vi "Medicao_anemometro.vi"(8 "Array 2":dbl[](array[numeric]), 9 "Sinalinp":dbl, 10 "Anemometro":dbl, 11 "DadosGraphInp":cluster{"GraphSenoide":i32[], "NivelAlto":bool}) -> (2 "Sinal":dbl, 3 "DadosGraph":cluster{"GraphSenoide":i32[], "NivelAlto":bool})   [LabVIEW 2019]
panel:
  out "Array":i32[](array[numeric])
  out "Anemometro 2":dbl
  in  "XY Graph 2":cluster{"X":dbl, "Y":dbl}[](graph)
  out "y 3":dbl
  out "y 2":dbl
  out "Array 4":dbl[](array[numeric])
  # "3,57812E+8"
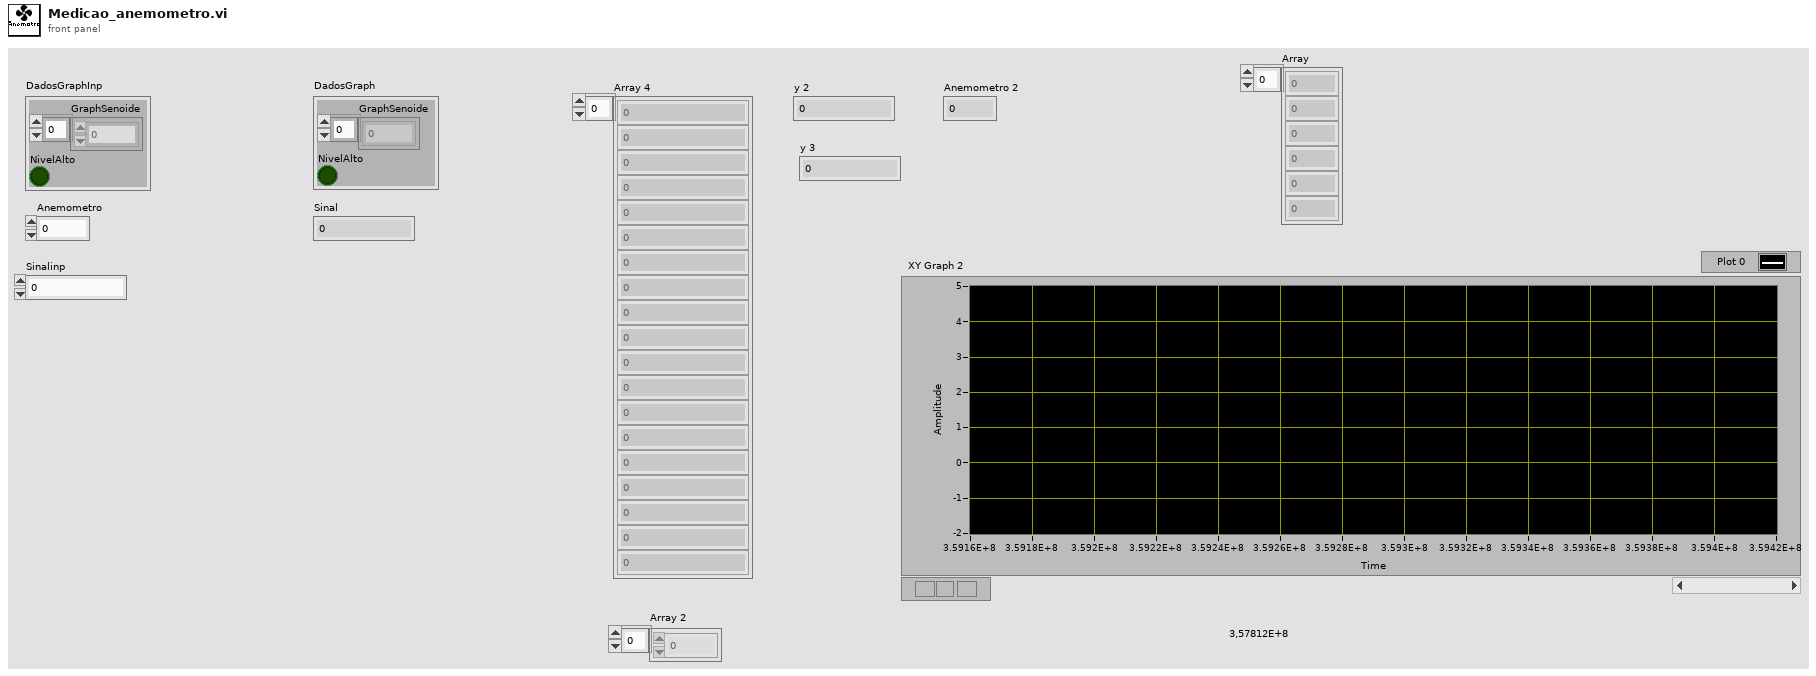
[diagram p1: front panel]
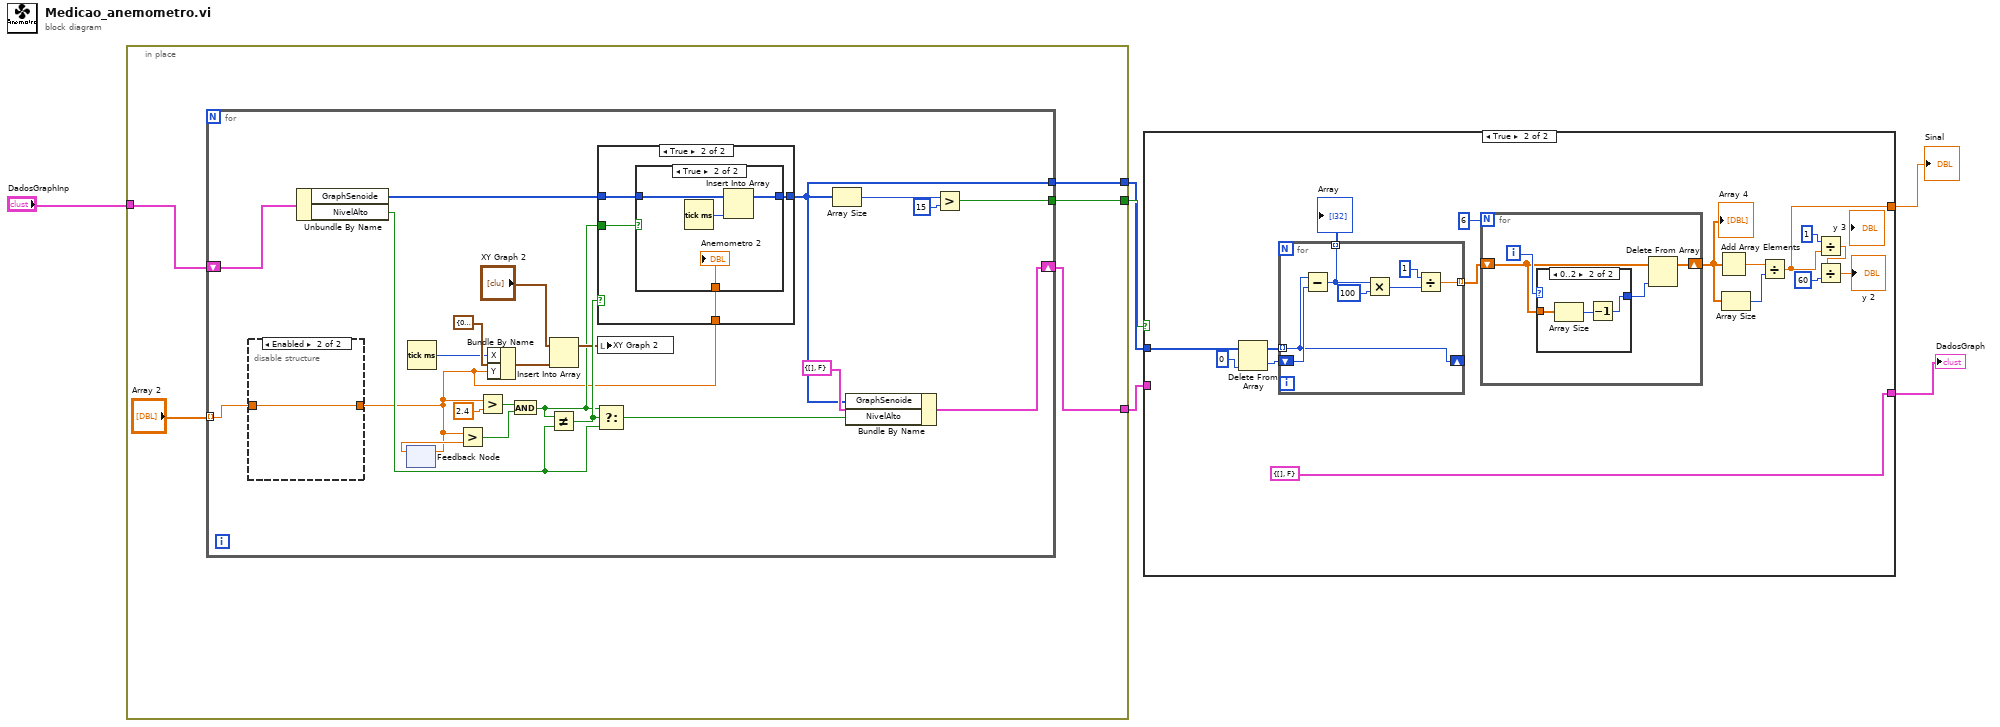
[diagram p0: block diagram]
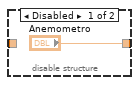
[diagram p2: hidden frame]
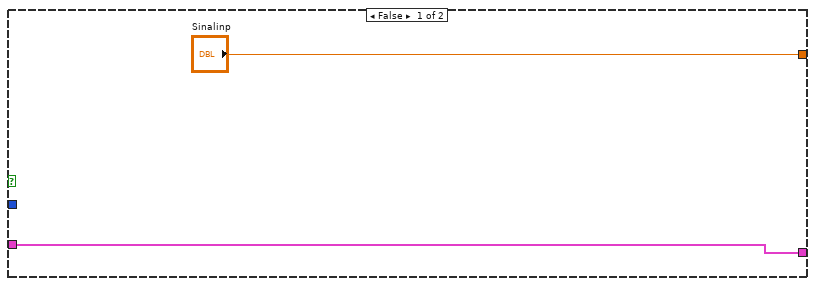
[diagram p5: hidden frame]
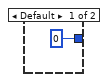
[diagram p6: hidden frame]
diagram:
  n1 = in-place {
    in-place-border: [w11] -> w6
    in-place-border: [w10] -> w5
    in-place-border: "DadosGraphInp" -> [w9]
    in-place-border: [w7] -> w3
    n2 = for {
      tunnel: [w34] -> w11
      tunnel: [w30] -> w10
      tunnel: "Array 2" -> [w13] mode=indexing
      shift-right: [w12] -> w7
      shift-left: w9 -> [w24]
      n3 = disable-structure shown="Enabled" {
        disable-tunnel: ["Anemometro" w36] -> w14
        disable-tunnel: w13 -> [_ w36]
        frame Disabled {
        }
        frame Enabled {
        }
      }
      n4 = Unbundle By Name(w24) -> ("GraphSenoide"=w33:i32[], "NivelAlto"=w32:bool)
      n5 = feedback #1() -> (w18:dbl)  [unwired: 1 in]
      n6 = feedback-in #1(w14) -> ()
      n7 = Tick Count (ms)() -> (millisecond timer value=w19:u32)
      n8 = Greater?(x=w14, y=w18) -> (0:w16:bool)
      n9 = Greater?(x=w14, y=2.4) -> (0:w17:bool)
      n10 = Bundle By Name(cluster=cluster{"X":dbl, "Y":dbl} {"X"=0.0, "Y"=0.0} ("new element/subarray"), "X"=w19, "Y"=w14) -> (w20:cluster{"X":dbl, "Y":dbl})
      n11 = And(x=w17, y=w16) -> (x .and. y?=w15:bool)
      n12 = Not Equal?(x=w15, y=w32) -> (x != y?=w26:bool)
      n13 = Insert Into Array(array="XY Graph 2", new element=w20) -> (w22:cluster{"X":dbl, "Y":dbl}[])  [unwired: 1 in]
      n14 = Select(t=w15, s=w26, f=w32) -> (s? t:f=w29:bool)
      n15 = case shown="True" w26 {
        tunnel: w33 -> [w37 w41]
        tunnel: [w37 w40] -> w30
        tunnel: w15 -> [_ w39]
        tunnel: w14 -> [_ w38]
        frame False {
        }
        frame True {
          n16 = case shown="True" w39 {
            tunnel: w41 -> [w42 w46]
            tunnel: [w42 w44] -> w40
            tunnel: w38 -> [_ w43]
            frame False {
            }
            frame True {
              n17 = Tick Count (ms)() -> (millisecond timer value=w45:u32)
              n18 = Insert Into Array(array=w46, new element=w45) -> (w44:i32[])  [unwired: 1 in]
              "Anemometro 2" <- w43
            }
          }
        }
      }
      n19 = local write "XY Graph 2"(w22) -> ()
      n20 = Array Size(array=w30) -> (size(s)=w28:i32)
      n21 = Bundle By Name(cluster=cluster{"GraphSenoide":i32[], "NivelAlto":bool} {"GraphSenoide"=[], "NivelAlto"=FALSE} ("DadosGraph"), "GraphSenoide"=w30, "NivelAlto"=w29) -> (w12:cluster{"GraphSenoide":i32[], "NivelAlto":bool})
      n22 = Greater?(x=w28, y=15) -> (0:w34:bool)
    }
  }
  n23 = case shown="True" w6 {
    tunnel: w5 -> [_ w64]
    tunnel: w3 -> [w48 _]
    tunnel: [w48 cluster{"GraphSenoide":i32[], "NivelAlto":bool} {"GraphSenoide"=[], "NivelAlto"=FALSE} ("DadosGraph")] -> w2
    tunnel: ["Sinalinp" w51] -> w1
    frame False {
    }
    frame True {
      n24 = Delete From Array(array=w64, index=0) -> (deleted portion=w62:i32, array with subset deleted=w61:i32[])  [unwired: 1 in]
      n25 = for {
        tunnel: w61 -> [w78] mode=indexing
        shift-right: [w78] -> _
        shift-left: w62 -> [w79]
        tunnel: [w76] -> w59 mode=indexing
        tunnel: [w73] -> w49 mode=indexing
        n26 = Subtract(x=w78, y=w79) -> (x-y=w73:i32)
        n27 = Multiply(x=w73, y=100) -> (x*y=w75:i32)
        n28 = Divide(x=1, y=w75) -> (x/y=w76:dbl)
      }
      "Array" <- w49
      n29 = for {
        N: 6 -> [_]
        shift-right: [w65] -> w57
        shift-left: w59 -> [w66]
        i -> [w67]
        n30 = case shown="0..2" w67 {
          tunnel: [0 w72] -> w68
          tunnel: w66 -> [_ w70]
          frame Default {
          }
          frame 0..2 {
            n31 = Array Size(array=w70) -> (size(s)=w71:i32)
            n32 = Decrement(x=w71) -> (x-1=w72:i32)
          }
        }
        n33 = Delete From Array(array=w66, index=w68) -> (array with subset deleted=w65:dbl[])  [unwired: 1 in, 1 out]
      }
      "Array 4" <- w57
      n34 = Add Array Elements(numeric array=w57) -> (sum=w58:dbl)
      n35 = Array Size(array=w57) -> (size(s)=w56:i32)
      n36 = Divide(x=w58, y=w56) -> (x/y=w51:dbl)
      n37 = Divide(x=1 ("index"), y=w51) -> (x/y=w50:dbl)
      n38 = Divide(x=w50, y=60 ("index")) -> (x/y=→"y 2":dbl)
    }
  }
  "DadosGraph" <- w2
  "Sinal" <- w1
